vi "FittingRange.vi"(0 "Array in (X)":i32[](array[numeric]), 1 "L0 DAC":i32, 2 "IPR":i32, 3 "upper limit":dbl=0.8, 5 "Array in (Y)":i32[](array[numeric]), 7 "Array Pointer in":i32, 9 "Cycles Burst":i32=10000, 11 "error in":errorcluster, 12 "State machine":i32, 13 "lower limit":dbl=0.2) -> (4 "Array out (X)":i32[](array[numeric]), 6 "Array out (Y)":i32[](array[numeric]), 8 "Array Pointer out":i32, 10 "N_Array Elements":i32, 14 "State machine":i32, 15 "error out":errorcluster)   [LabVIEW 2009]
doc: "This VI collects the L0 DAC values that gives an IPR between the 80%-20% of the generated pulses."
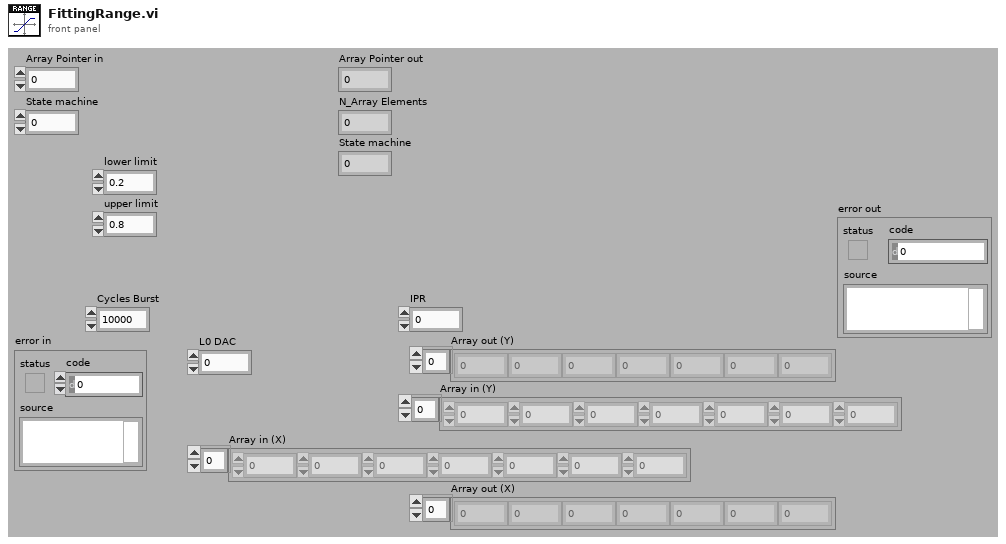
[diagram p1: front panel]
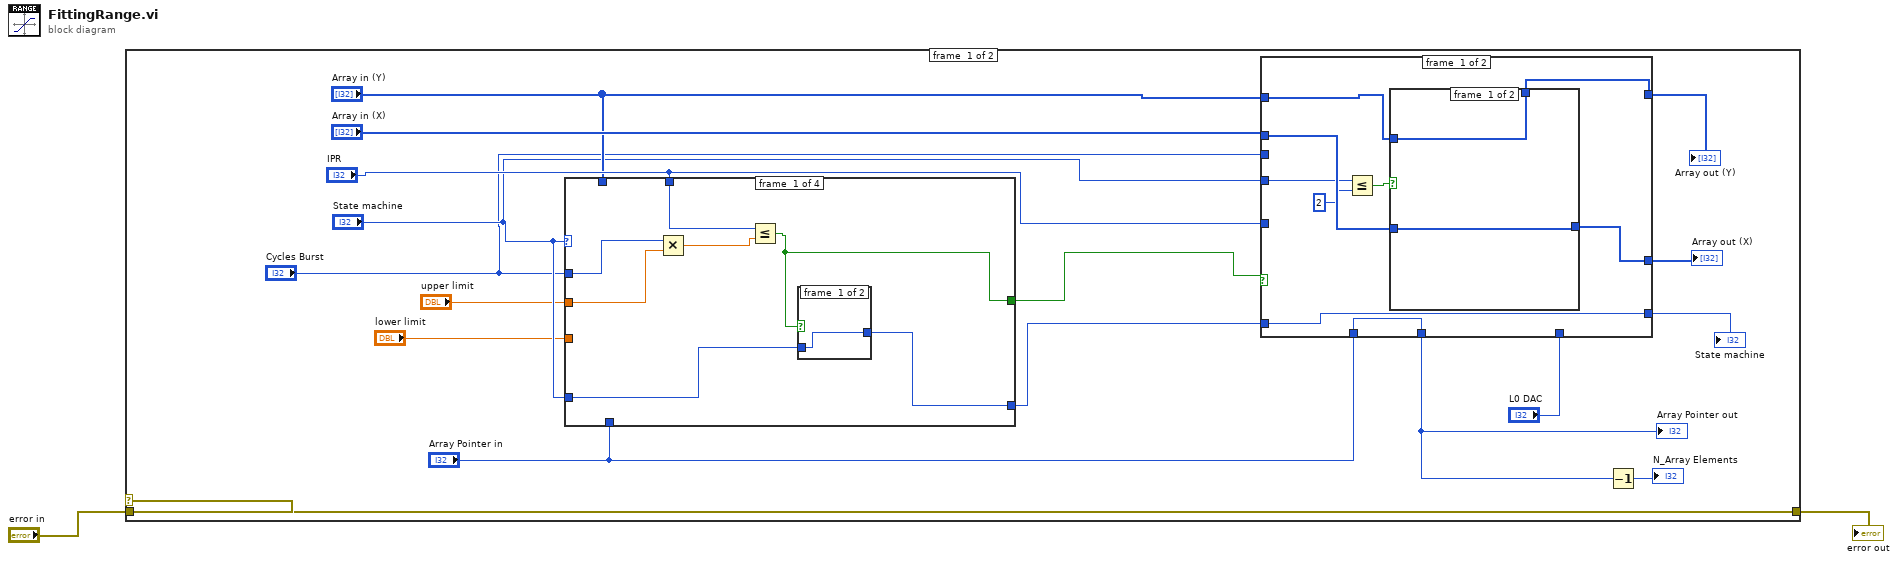
[diagram p0: block diagram]
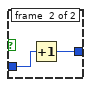
[diagram p2: hidden frame]
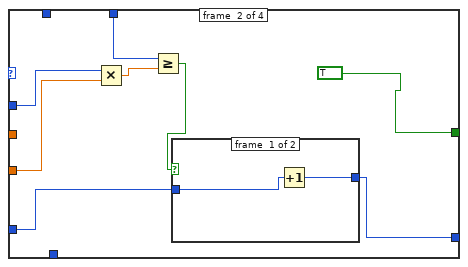
[diagram p3: hidden frame]
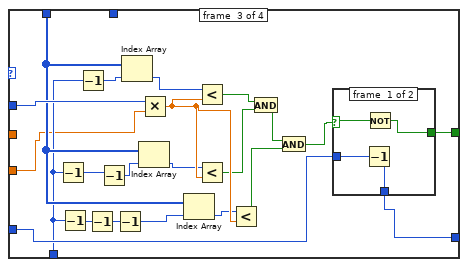
[diagram p5: hidden frame]
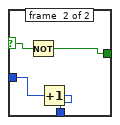
[diagram p6: hidden frame]
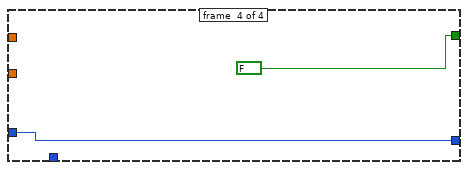
[diagram p7: hidden frame]
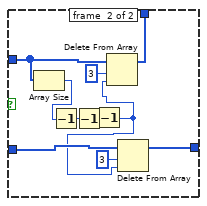
[diagram p8: hidden frame]
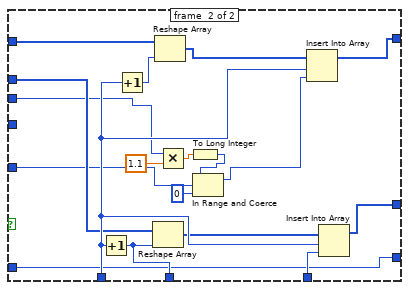
[diagram p9: hidden frame]
diagram:
  n1 = case shown="No Error" "error in" {
    tunnel: "error in" -> [w15 w112]
    tunnel: [w15 w112] -> w1
    frame #0 {
      n2 = case shown="1" "State machine" {
        tunnel: "Cycles Burst" -> [w25 w31 w62 _]
        tunnel: "IPR" -> [w24 w30 _ _]
        tunnel: "State machine" -> [w23 w35 w49 w72]
        tunnel: [w22 w36 w50 w72] -> w9
        tunnel: "Array in (Y)" -> [_ _ w59 _]
        tunnel: "Array Pointer in" -> [_ _ w44 _]
        tunnel: [w21 TRUE w42 FALSE ("record")] -> w6
        tunnel: "lower limit" -> [_ w32 w41 _]
        tunnel: "upper limit" -> [w20 _ _ _]
        frame #0 {
          n3 = Multiply(x=w25, y=w20) -> (x*y=w26:dbl)
          n4 = Less Or Equal?(x=w24, y=w26) -> (x <= y?=w21:bool)
          n5 = case shown="False" w21 {
            tunnel: w23 -> [w27 w29]
            tunnel: [w27 w28] -> w22
            frame #0 {
            }
            frame #1 {
              n6 = Increment(x=w29) -> (x+1=w28:i32)
            }
          }
        }
        frame #1 {
          n7 = Multiply(x=w31, y=w32) -> (x*y=w37:dbl)
          n8 = Greater Or Equal?(x=w30, y=w37) -> (x >= y?=w34:bool)
          n9 = case shown="True" w34 {
            tunnel: [w39 w40] -> w36
            tunnel: w35 -> [w38 w40]
            frame #0 {
              n10 = Increment(x=w38) -> (x+1=w39:i32)
            }
            frame #1 {
            }
          }
        }
        frame #2 {
          n11 = Decrement(x=w44) -> (x-1=w46:i32)
          n12 = Decrement(x=w44) -> (x-1=w58:i32)
          n13 = Decrement(x=w44) -> (x-1=w43:i32)
          n14 = Decrement(x=w58) -> (x-1=w48:i32)
          n15 = Decrement(x=w46) -> (x-1=w45:i32)
          n16 = Decrement(x=w48) -> (x-1=w47:i32)
          n17 = Index Array(array=w59, index=w43) -> (element=w61:i32)
          n18 = Index Array(array=w59, index=w45) -> (element=w55:i32)
          n19 = Multiply(x=w62, y=w41) -> (x*y=w57:dbl)
          n20 = Index Array(array=w59, index=w47) -> (element=w56:i32)
          n21 = Less?(x=w61, y=w57) -> (x < y?=w60:bool)
          n22 = Less?(x=w55, y=w57) -> (x < y?=w54:bool)
          n23 = Less?(x=w56, y=w57) -> (x < y?=w52:bool)
          n24 = And(x=w60, y=w54) -> (x .and. y?=w53:bool)
          n25 = And(x=w53, y=w52) -> (x .and. y?=w51:bool)
          n26 = case shown="True" w51 {
            selector: w51 -> [w63 w67]
            tunnel: [w66 w70] -> w50
            tunnel: w49 -> [w65 w69]
            tunnel: [w64 w68] -> w42
            frame #0 {
              n27 = Decrement(x=w65) -> (x-1=w66:i32)
              n28 = Not(x=w63) -> (.not. x?=w64:bool)
            }
            frame #1 {
              n29 = Not(x=w67) -> (.not. x?=w68:bool)
              n30 = Increment(x=w69) -> (x+1=w70:i32)
            }
          }
        }
        frame #3 {
        }
      }
      n31 = case shown="True" w6 {
        tunnel: "IPR" -> [_ w100]
        tunnel: [w78 w106] -> w19
        tunnel: "Array in (Y)" -> [w79 w108]
        tunnel: "L0 DAC" -> [_ w111]
        tunnel: "Array in (X)" -> [w76 w102]
        tunnel: [w77 w103] -> w16
        tunnel: "Array Pointer in" -> [w81 w105]
        tunnel: [w81 w109] -> w13
        tunnel: w9 -> [w80 w101]
        tunnel: [w80 w101] -> w8
        tunnel: "State machine" -> [w74 _]
        tunnel: "Cycles Burst" -> [_ w96]
        frame #0 {
          n32 = Less Or Equal?(x=w74, y=2) -> (x <= y?=w75:bool)
          n33 = case shown="True" w75 {
            tunnel: w79 -> [w83 w93]
            tunnel: [w83 w88] -> w78
            tunnel: [w82 w86] -> w77
            tunnel: w76 -> [w82 w85]
            frame #0 {
            }
            frame #1 {
              n34 = Array Size(array=w93) -> (size(s)=w92:i32)
              n35 = Decrement(x=w92) -> (x-1=w91:i32)
              n36 = Decrement(x=w91) -> (x-1=w90:i32)
              n37 = Decrement(x=w90) -> (x-1=w84:i32)
              n38 = Delete From Array(array=w93, length=3, index=w84) -> (array with subset deleted=w88:i32[])  [unwired: 1 out]
              n39 = Delete From Array(array=w85, length=3, index=w84) -> (array with subset deleted=w86:i32[])  [unwired: 1 out]
            }
          }
        }
        frame #1 {
          n40 = Increment(x=w105) -> (x+1=w109:i32)
          n41 = Increment(x=w105) -> (x+1=w110:i32)
          n42 = Reshape Array(w102, w109) -> (w104:i32[])
          n43 = Reshape Array(w108, w110) -> (w107:i32[])
          n44 = Multiply(x=w96, y=1.1) -> (x*y=w95:dbl)
          n45 = To Long Integer(number=w95) -> (32bit integer=w94:i32)
          n46 = In Range and Coerce(upper limit=w94, x=w100, lower limit=0) -> (coerced(x)=w99:i32)  [unwired: 1 out]
          n47 = Insert Into Array(array=w107, index=w105, new element=w99) -> (w106:i32[])
          n48 = Insert Into Array(array=w104, index=w105, new element=w111) -> (w103:i32[])
        }
      }
      "Array out (Y)" <- w19
      "Array out (X)" <- w16
      "Array Pointer out" <- w13
      "State machine" <- w8
      n49 = Decrement(x=w13) -> (x-1=→"N_Array Elements":i32)
    }
    frame #1 {
    }
  }
  "error out" <- w1
